vi "File.Move to Archive Folder.vi"(6 "NameSuffix":string, 8 "error in (no error)":errorcluster, 9 "SubDirList":string[](array[string]) caption="Opt - SubDir List", 10 "ArchiveDir":path, 11 "UUTDir":path) -> (0 "error out":errorcluster, 2 "Archived":bool)   [LabVIEW 2024]
uses:
  Errors/Error.Error Code List.ctl
  Errors.lvlib
  File Utils.lvlib
panel:
  out "Path":path
  # "If not archived and no error then was empty"
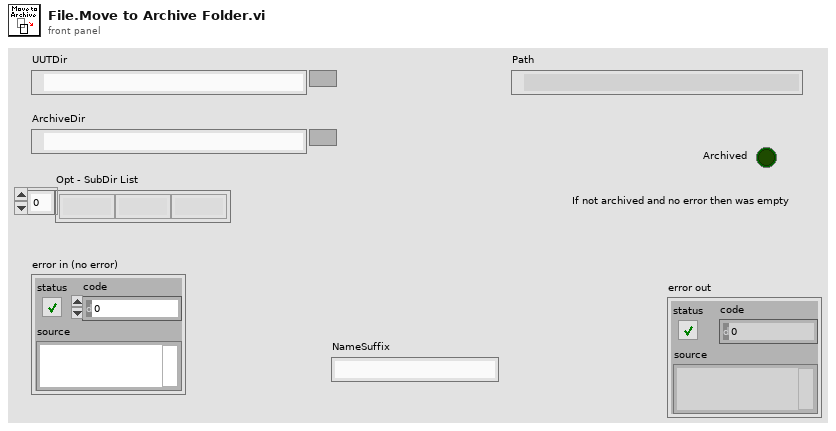
[diagram p1: front panel]
types:
  T1 = cluster{"UUTDir":path, "ArchiveDir":path, "DestDir":path, "SubDirList":string[], "Archived":bool, "NameSuffix":string}
  T2 = typedef "EQMF.lvlib/Errors.lvlib/Error.Error Code List.ctl" = i32
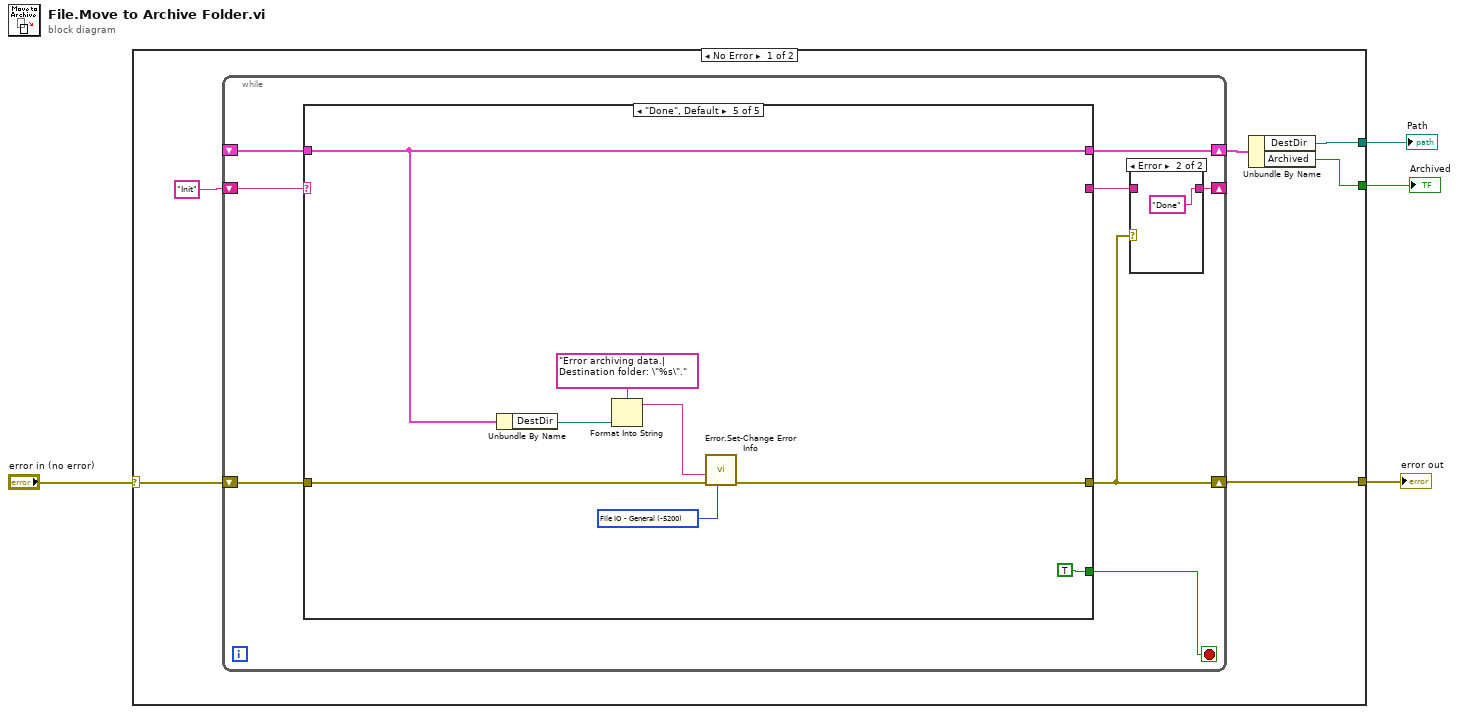
[diagram p0: block diagram]
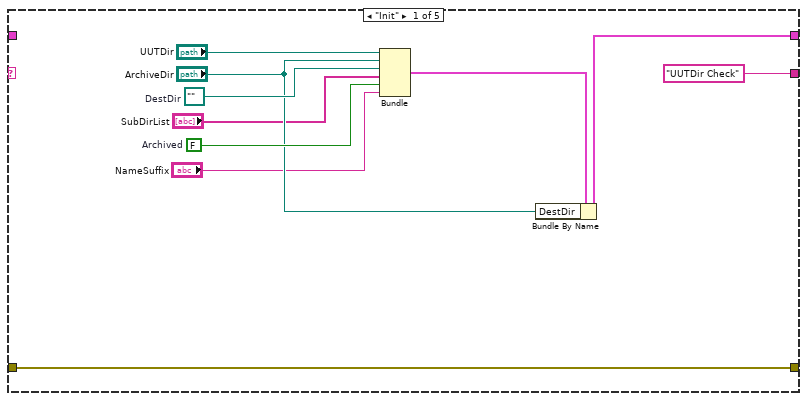
[diagram p3: hidden frame]
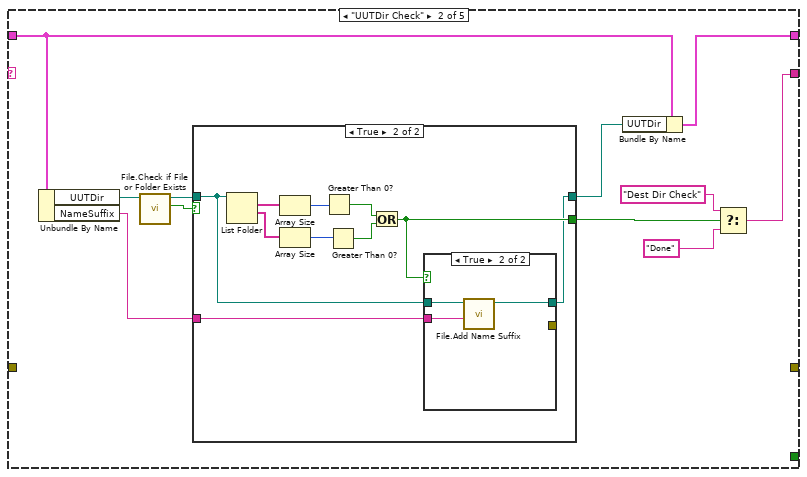
[diagram p4: hidden frame]
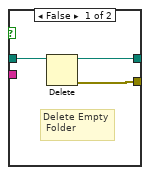
[diagram p6: hidden frame]
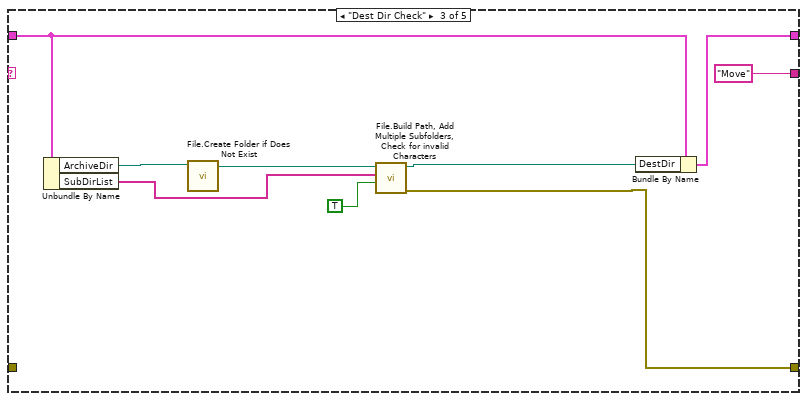
[diagram p7: hidden frame]
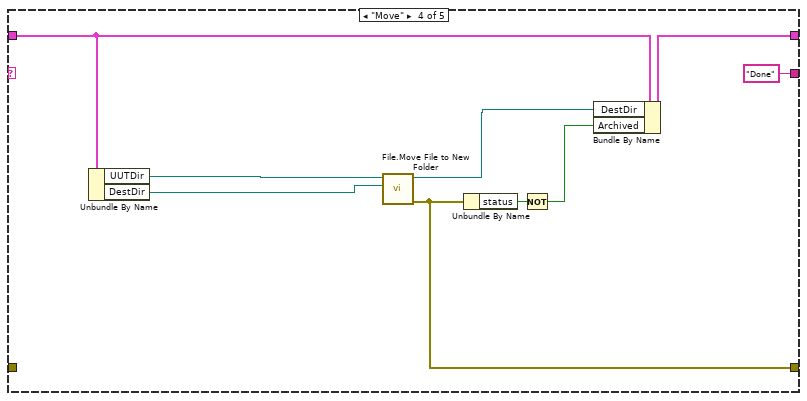
[diagram p8: hidden frame]
diagram:
  n1 = case shown="No Error" "error in (no error)" {
    selector: "error in (no error)" -> [w10 _]
    tunnel: [w5 _] -> w3
    tunnel: [w7 _] -> w2
    tunnel: [w6 _] -> w1
    frame No Error {
      n2 = while {
        shift-right: [w18] -> w8
        shift-left: _ -> [w16]
        shift-right: [w13] -> w5
        shift-left: w10 -> [w15]
        shift-right: [w11] -> _
        shift-left: "Init" -> [w17]
        stop <- w14 stop-if-true
        n3 = case shown="\"Done\", Default" w17 {
          tunnel: [w25 w31 w64 w76 w78] -> w18
          tunnel: ["UUTDir Check" w36 "Move" "Done" _] -> w12
          tunnel: w16 -> [_ w32 w65 w75 w78]
          tunnel: w15 -> [w28 _ _ _ w80]
          tunnel: [w28 _ w59 w71 w79] -> w13
          tunnel: [_ _ _ _ TRUE] -> w14
          frame "Init" {
            w24 = FALSE  # Archived
            w27 = path ""  # DestDir
            n4 = Bundle("UUTDir"="UUTDir", "ArchiveDir"="ArchiveDir", "DestDir"=w27, "SubDirList"="SubDirList", "Archived"=w24, "NameSuffix"="NameSuffix") -> (w26:T1)  [unwired: 1 in]
            n5 = Bundle By Name(cluster=w26, "DestDir"="ArchiveDir") -> (w25:T1)
          }
          frame "UUTDir Check" {
            n6 = Unbundle By Name(w32) -> ("UUTDir"=w41:path, "NameSuffix"=w34:string)
            n7 = call "File.Check if File or Folder Exists.vi"("Path"=w41) -> ("Exists"=w39:bool, "Dup Path"=w40:path)  [unwired: 6 in, 3 out]
            n8 = case shown="True" w39 {
              tunnel: w40 -> [w42 w46]
              tunnel: [_ w45] -> w35
              tunnel: w34 -> [_ w44]
              tunnel: [w42 w43] -> w33
              frame False {
              }
              frame True {
                n9 = List Folder(path=w46) -> (filenames=w52:string[], folder names=w51:string[])  [unwired: 3 in, 2 out]
                n10 = Array Size(array=w52) -> (size(s)=w50:i32)
                n11 = Array Size(array=w51) -> (size(s)=w49:i32)
                n12 = Greater Than 0?(x=w50) -> (x > 0?=w47:bool)
                n13 = Greater Than 0?(x=w49) -> (x > 0?=w48:bool)
                n14 = Or(x=w47, y=w48) -> (x .or. y?=w45:bool)
                n15 = case shown="True" w45 {
                  tunnel: w46 -> [w55 w58]
                  tunnel: [w54 _] -> _
                  tunnel: w44 -> [_ w57]
                  tunnel: [w53 w56] -> w43
                  frame False {
                    # "Delete Empty\n Folder"
                    n16 = Delete(path (use dialog)=w55) -> (deleted path=w53:path, error out=w54:errorcluster)  [unwired: 4 in, 1 out]
                  }
                  frame True {
                    n17 = call "File.Add Name Suffix.vi"("Suffix"=w57, "Source"=w58) -> ("New Path"=w56:path)  [unwired: 8 in, 1 out]
                  }
                }
              }
            }
            n18 = Bundle By Name(cluster=w32, "UUTDir"=w33) -> (w31:T1)
            n19 = Select(t="Dest Dir Check", s=w35, f="Done") -> (s? t:f=w36:string)
          }
          frame "Dest Dir Check" {
            n20 = Unbundle By Name(w65) -> ("ArchiveDir"=w66:path, "SubDirList"=w61:string[])
            n21 = call "File.Create Folder if Does Not Exist.vi"("Path"=w66) -> ("Dup Path"=w62:path)  [unwired: 8 in, 2 out]
            n22 = call "File.Build Path, Add Multiple Subfolders, Check for invalid Characters.vi"("Check/Create Dir"=TRUE, "Subfolders"=w61, "Folder"=w62) -> ("error out"=w59:errorcluster, "New Path"=w60:path)  [unwired: 6 in, 1 out]
            n23 = Bundle By Name(cluster=w65, "DestDir"=w60) -> (w64:T1)
          }
          frame "Move" {
            n24 = Unbundle By Name(w75) -> ("UUTDir"=w74:path, "DestDir"=w73:path)
            n25 = call "File.Move File to New Folder.vi"("Destination Folder"=w73, "Source File Path"=w74) -> ("error out"=w71:errorcluster, "New Path"=w72:path)  [unwired: 8 in]
            n26 = Unbundle By Name(w71) -> ("status"=w70:bool)
            n27 = Not(x=w70) -> (.not. x?=w69:bool)
            n28 = Bundle By Name(cluster=w75, "DestDir"=w72, "Archived"=w69) -> (w76:T1)
          }
          frame "Done", Default {
            w83 = T2 -5200 items=["No Error"=0, "Abort"=-2, "Misc"=-5000, "Fixture Error"=-5100, "File IO - General"=-5200, "FIle IO - Config Error"=-5201, "Instrument - General"=-5300, "Instrument - Serial Com"=-5301, "Instrument - Camera"=-5302, "Instrument - PS"=-5303, "Instrument - Oscilloscope"=-5304, "Instrument - Function Gen"=-5305, "Instrument - Load"=-5306, "Instrument - Meter"=-5307, "Instrument - Power Control"=-5308, "Instrument - Motion"=-5309, "Instrument - RF"=-5310, "System Exe"=-5400, "Image Processing"=-5500, "Communication"=-5600, "Script - Syntax Error"=-6000, "Script - Invalid Name or Param"=-6100, "Script - Timeout"=-6200, "Invalid Data"=-6300, "FW Update Error"=-6500] ("Std Code")
            n29 = Unbundle By Name(w78) -> ("DestDir"=w77:path)
            n30 = Format Into String(format string="Error archiving data.| Destination folder: \"%s\".", w77) -> (resulting string=w81:string)  [unwired: 2 in, 1 out]
            n31 = call "Error.Set-Change Error Info.vi"("Std Code"=w83, "error in"=w80, "Description"=w81) -> ("error out"=w79:errorcluster)  [unwired: 8 in]
          }
        }
        n32 = case shown="Error" w13 {
          tunnel: w12 -> [w19 _]
          tunnel: [w19 "Done"] -> w11
          frame No Error {
          }
          frame Error {
          }
        }
      }
      n33 = Unbundle By Name(w8) -> ("DestDir"=w7:path, "Archived"=w6:bool)
    }
    frame Error {
    }
  }
  "error out" <- w3
  "Path" <- w2
  "Archived" <- w1
